vi "BRig_dataCurrent_RunTime.vi"() -> (2 "output_RunTime":i32)   [LabVIEW 2014]
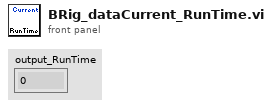
[diagram p1: front panel]
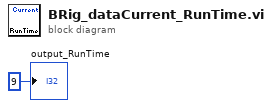
[diagram p0: block diagram]
diagram:
  "output_RunTime" <- 9 ("output_iBlock")
